vi "Identify.vi"(8 "error in (no error)":errorcluster, 11 "Servo to Power Out in":refnum<class "Servo to Power Out.lvclass">) -> (0 "error out":errorcluster, 2 "Plugin is Valid":bool, 3 "Servo to Power Out out":refnum<class "Servo to Power Out.lvclass">)   [LabVIEW 2018, in "Servo to Power Out.lvlib" / "Servo to Power Out.lvclass"]
uses:
  Servo to Power Out.lvclass
  C:/Sequence Automation/Plugins/Measurement Interface.lvlibp/Measurement Interface.lvclass
  Plugins/Measurement Interface.lvlibp/Private Methods/Measurement Definition Entry/Read Measurement Definition Entry.vi
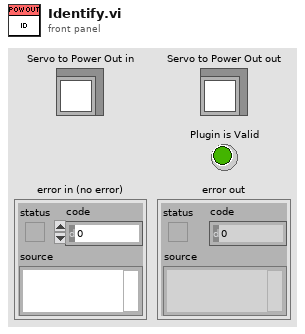
[diagram p1: front panel]
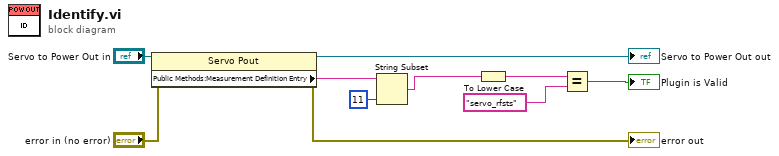
[diagram p0: block diagram]
diagram:
  n1 = property class="Servo Pout"(reference="Servo to Power Out in", error in="error in (no error)") -> (reference out=→"Servo to Power Out out":refnum<class "Servo to Power Out.lvclass">, error out=→"error out":errorcluster, "Public Methods:Measurement Definition Entry"=w5:string)
  n2 = String Subset(string=w5, length (rest)=11 ("length (rest)")) -> (substring=w3:string)  [unwired: 1 in]
  n3 = To Lower Case(string=w3) -> (all lower case string=w2:string)
  n4 = Equal?(x=w2, y="servo_rfsts") -> (x = y?=→"Plugin is Valid":bool)
